vi "Driver Update Table for Spartan 5.0.vi"(8 "error in (no error)":errorcluster, 11 "Connection Refnum":T1) -> (0 "error out":errorcluster, 3 "dup Connection Refnum":T1)   [LabVIEW 2011]
uses:
  Summitek EXT/ODBC/SQL Controls/Connection Refnum.ctl
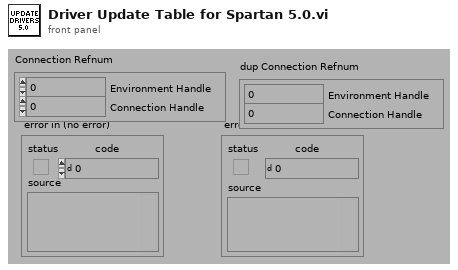
[diagram p1: front panel]
types:
  T1 = typedef "Connection Refnum.ctl" = cluster{"Environment Handle":i32, "Connection Handle":i32}
  T2 = typedef "Statement Refnum.ctl" = cluster{"Statement Handle":i32, "Parameter Number":u16}
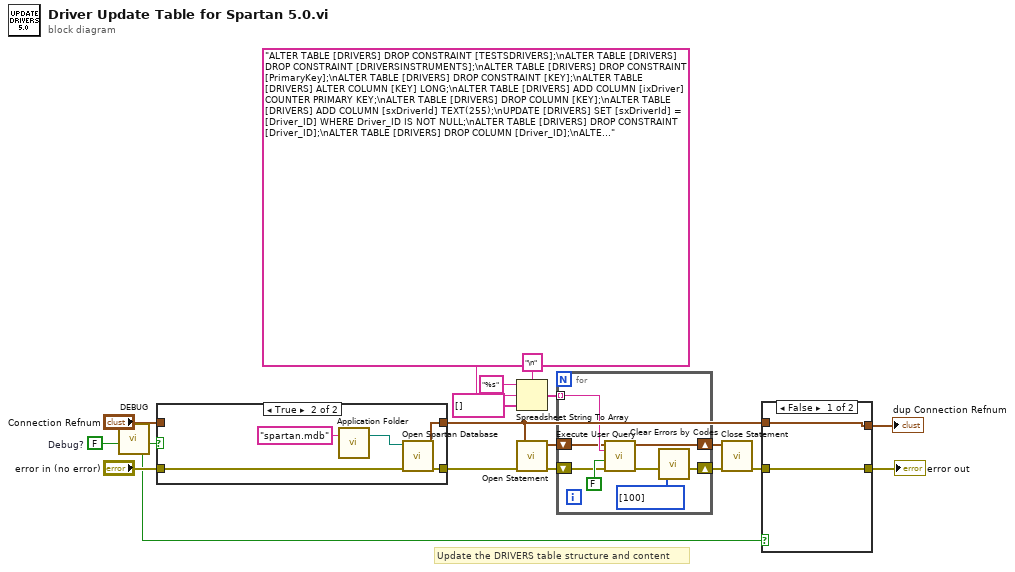
[diagram p0: block diagram]
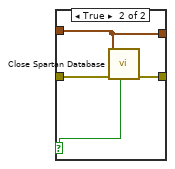
[diagram p3: hidden frame]
diagram:
  w6 = FALSE  # Debug?
  # "Update the DRIVERS table structure and content"
  n1 = call "DEBUG.vi"("Dev DEBUG? (f)"=w6) -> ("DEBUG?"=w5:bool)  [unwired: 1 in, 5 out]
  n2 = case shown="True" w5 {
    tunnel: "Connection Refnum" -> [w20 _]
    tunnel: "error in (no error)" -> [w19 w25]
    tunnel: [w19 w24] -> w7
    tunnel: [w20 w23] -> w3
    frame False {
    }
    frame True {
      n3 = call "Application Folder.vi"("Relative Path (\"\" - Folder)"="spartan.mdb" ("Relative Path (\"\" - Folder)")) -> ("Application Folder"=w21:path)  [unwired: 2 in]
      n4 = call "Open Spartan Database.vi"("error in (no error)"=w25, "DB Path (empty - use default)"=w21) -> ("error out"=w24:errorcluster, "Connection Refnum"=w23:T1)  [unwired: 1 in, 7 out]
    }
  }
  n5 = Spreadsheet String To Array(delimiter (Tab)="\n", format string="%s", spreadsheet string="ALTER TABLE [DRIVERS] DROP CONSTRAINT [TESTSDRIVERS];\nALTER TABLE [DRIVERS] DROP CONSTRAINT [DRIVERSINSTRUMENTS];\nALTER TABLE [DRIVERS] DROP CONSTRAINT [PrimaryKey];\nALTER TABLE [DRIVERS] DROP CONSTRAINT [KEY];\nALTER TABLE [DRIVERS] ALTER COLUMN [KEY] LONG;\nALTER TABLE [DRIVERS] ADD COLUMN [ixDriver] COUNTER PRIMARY KEY;\nALTER TABLE [DRIVERS] DROP COLUMN [KEY];\nALTER TABLE [DRIVERS] ADD COLUMN [sxDriverId] TEXT(255);\nUPDATE [DRIVERS] SET [sxDriverId] = [Driver_ID] WHERE Driver_ID IS NOT NULL;\nALTER TABLE [DRIVERS] DROP CONSTRAINT [Driver_ID];\nALTER TABLE [DRIVERS] DROP COLUMN [Driver_ID];\nALTER TABLE [DRIVERS] ADD COLUMN [sType] TEXT(255);\nUPDATE [DRIVERS] SET [sType] = [DriverType];\nALTER TABLE [DRIVERS] DROP COLUMN [DriverType]; \nALTER TABLE [DRIVERS] ADD COLUMN [sVersion] TEXT(255);\nALTER TABLE [DRIVERS] ADD COLUMN [sTemp] TEXT(255);\nUPDATE [DRIVERS] SET [sTemp] = [Build];\nALTER TABLE [DRIVERS] DROP COLUMN [Build];\nUPDATE [DRIVERS] SET [sVersion] = [Version]+'.'+[sTemp];\nALTER TABLE [DRIVERS] DROP COLUMN [sTemp];\nALTER TABLE [DRIVERS] DROP COLUMN [Version];" ("User Query"), array type (2D Dbl)=string[] []) -> (array=w17:string[])
  n6 = call "Open Statement.vi"("error in (no error)"=w7, "Connection Refnum"=w3) -> ("error out"=w14:errorcluster, "Statement Refnum"=w13:T2)  [unwired: 4 out]
  n7 = for {
    shift-right: [w26] -> w12
    shift-left: w14 -> [w30]
    tunnel: w17 -> [w32] mode=indexing
    shift-right: [w29] -> w11
    shift-left: w13 -> [w31]
    n8 = call "Execute User Query.vi"("error in (no error)"=w30, "Return Data? (f)"=FALSE, "User Query"=w32, "Statement Refnum"=w31) -> ("error out"=w27:errorcluster, "Statement Refnum"=w29:T2)  [unwired: 2 out]
    n9 = call "Clear Errors by Codes.vi"("Error Codes\nto Clear (Empty)"=i32[] [100] ("Error Codes\nto Clear (Empty)"), "error in (no error)"=w27) -> ("error out"=w26:errorcluster)  [unwired: 5 out]
  }
  n10 = call "Close Statement.vi"("error in (no error)"=w12, "Statement Refnum"=w11) -> ("error out"=w4:errorcluster)  [unwired: 5 out]
  n11 = case shown="False" w5 {
    selector: w5 -> [_ w37]
    tunnel: w4 -> [w35 w39]
    tunnel: w3 -> [w34 w36]
    tunnel: [w35 w38] -> w10
    tunnel: [w34 w36] -> w1
    frame False {
    }
    frame True {
      n12 = call "Close Spartan Database.vi"("Force Close? (f)"=w37, "error in (no error)"=w39, "Connection Refnum"=w36) -> ("error out"=w38:errorcluster)  [unwired: 2 in, 6 out]
    }
  }
  "error out" <- w10
  "dup Connection Refnum" <- w1
